vi "6480-WaitInId.vi"(6 "time(0.1)":i32=100, 8 "error in":errorcluster, 9 "Wait?":bool=TRUE, 10 "Status":bool, 11 "IO_Input":T1) -> (0 "error Out":errorcluster, 2 "TimeOut":bool, 3 "StatusOut":bool)   [LabVIEW 2015]
uses:
  Ctrl/6480_SelectInPut.ctl
  Ctrl/IO Card_Type.ctl
  global/InAndOutGB.vi
  global/IO_FlagGB.vi
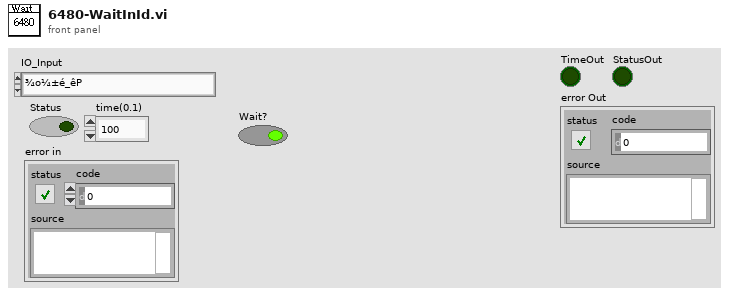
[diagram p1: front panel]
types:
  T1 = typedef "6480_SelectInPut.ctl" = enum16{"¾o¼±é_êP", "šâ‰º™zÖª", "¹â–Å#1", "¹â–Å#2", "¹â–Å#3", "ÉÏÏÂÁÏ™CReady", "ÉÏÏÂÁÏC¹ÊÕÏÓÌ", "ÉÏÏÂÁÏ™C¿ÉÎüÁÏ", "ÉÏÏÂÁÏ™C¿É·ÅPASS", "ÉÏÏÂÁÏ™C¿É·ÅNG1", "ÉÏÏÂÁÏ™C¿É·ÅNG2", "‚äÓÃ#2", "‚äÓÃ#3", "ñRß_µ½Î»ÓÌ"}
  T2 = typedef "IO Card_Type.ctl" = enum16{"None", "Unidaq32", "IPC_3005(9700)", "6480", "2410C-64", "Zan"}
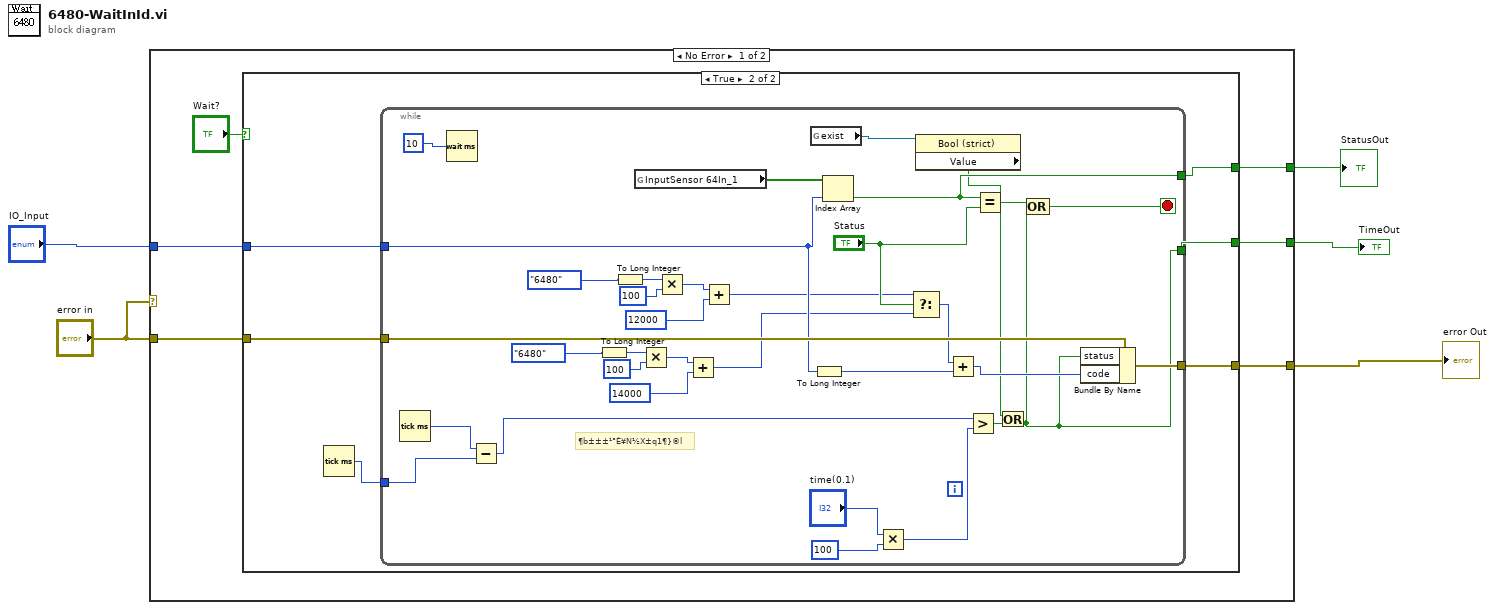
[diagram p0: block diagram]
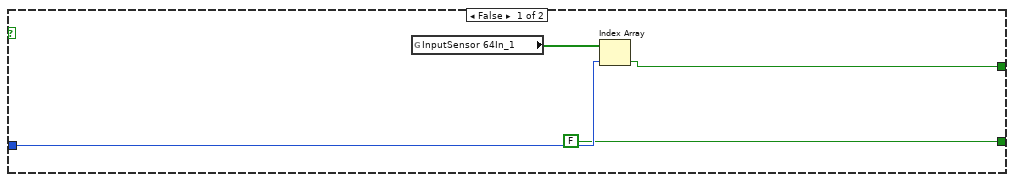
[diagram p2: hidden frame]
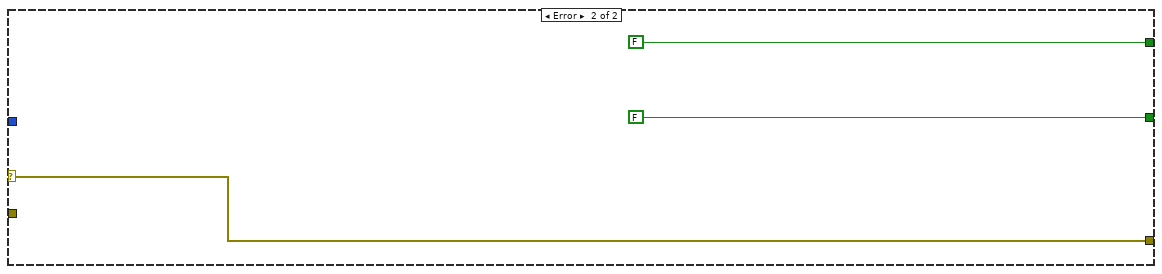
[diagram p3: hidden frame]
diagram:
  n1 = case shown="No Error" "error in" {
    selector: "error in" -> [_ w57]
    tunnel: [w11 FALSE] -> w5
    tunnel: "error in" -> [w10 _]
    tunnel: [w9 w57] -> w4
    tunnel: [w8 FALSE ("Boolean")] -> w2
    tunnel: "IO_Input" -> [w6 _]
    frame No Error {
      n2 = case shown="True" "Wait?" {
        tunnel: [FALSE w21] -> w11
        tunnel: w10 -> [_ w20]
        tunnel: [_ w19] -> w9
        tunnel: [w13 w18] -> w8
        tunnel: w6 -> [w14 w17]
        frame False {
          n3 = global read "InAndOutGB.vi" "InputSensor 64In_1"() -> (w15:bool[])
          n4 = Index Array(array=w15, index=w14) -> (element=w13:bool)
        }
        frame True {
          n5 = Tick Count (ms)() -> (millisecond timer value=w16:u32)
          n6 = while {
            tunnel: [w44] -> w21
            tunnel: w20 -> [w51]
            tunnel: [w48] -> w19
            tunnel: [w43] -> w18
            tunnel: w17 -> [w41]
            tunnel: w16 -> [w23]
            stop <- w53 stop-if-true
            # "¶b±±±¹°È¥N½X±q1¶}©l"
            n7 = Tick Count (ms)() -> (millisecond timer value=w24:u32)
            n8 = Wait (ms)(milliseconds to wait=u32 10) -> ()  [unwired: 1 out]
            n9 = Subtract(x=w24, y=w23) -> (x-y=w22:u32)
            n10 = To Long Integer(number=IO_Card_Type."6480" ("IO Card Type")) -> (32bit integer=w30:i32)
            n11 = To Long Integer(number=IO_Card_Type."6480" ("IO Card Type")) -> (32bit integer=w38:i32)
            n12 = global read "InAndOutGB.vi" "InputSensor 64In_1"() -> (w54:bool[])
            n13 = Multiply(x=w30, y=100) -> (x*y=w32:i32)
            n14 = Multiply(x=w38, y=100) -> (x*y=w36:i32)
            n15 = Add(x=w32, y=14000) -> (x+y=w28:i32)
            n16 = Add(x=w36, y=12000) -> (x+y=w34:i32)
            n17 = global read "IO_FlagGB.vi" "exist"() -> (w40:refnum<vi>)
            n18 = To Long Integer(number=w41) -> (32bit integer=w45:i32)
            n19 = Index Array(array=w54, index=w41) -> (element=w43:bool)
            n20 = Multiply(x="time(0.1)", y=u32 100 ("milliseconds to wait")) -> (x*y=w25:u32)
            n21 = Select(t=w34, s="Status", f=w28) -> (s? t:f=w46:i32)
            n22 = property class="Bool (strict)"(reference=w40) -> ("Value"=w42:bool)  [unwired: 1 in, 2 out]
            n23 = Add(x=w46, y=w45) -> (x+y=w49:i32)
            n24 = Greater?(x=w22, y=w25) -> (0:w50:bool)
            n25 = Equal?(x=w43, y="Status") -> (x = y?=w52:bool)
            n26 = Or(x=w42, y=w50) -> (x .or. y?=w44:bool)
            n27 = Compound Arithmetic op=OR(w52, w44) -> (w53:bool)
            n28 = Bundle By Name(cluster=w51, "status"=w44, "code"=w49) -> (w48:errorcluster)
          }
        }
      }
    }
    frame Error {
    }
  }
  "TimeOut" <- w5
  "error Out" <- w4
  "StatusOut" <- w2
